vi "Hi-Tec_calibs.vi"(5 "Gas Line Name":string) -> (1 "Hi-Tec calib":T1={"Ref temp (deg C)"=0.0, "Ref Pres (mbars)"=0.0, "Density at calib conditions"=-0.0141, "Coefficients"=[]} {"Coefficients" format="%.2f"; "Density at calib conditions" format="%.4f"; "Ref Pres (mbars)" format="%.2f"; "Ref temp (deg C)" format="%.2f"}, 2 "Comments":string)   [LabVIEW 2015]
uses:
  Controls/Hi-Tec_calib.ctl
  Anemometry/Anemometry Sub Vis/Globals/Gas_management_global.vi
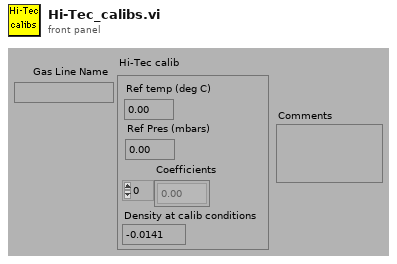
[diagram p1: front panel]
types:
  T1 = typedef "Hi-Tec_calib.ctl" = cluster{"Ref temp (deg C)":dbl, "Ref Pres (mbars)":dbl, "Density at calib conditions":dbl, "Coefficients":dbl[]}
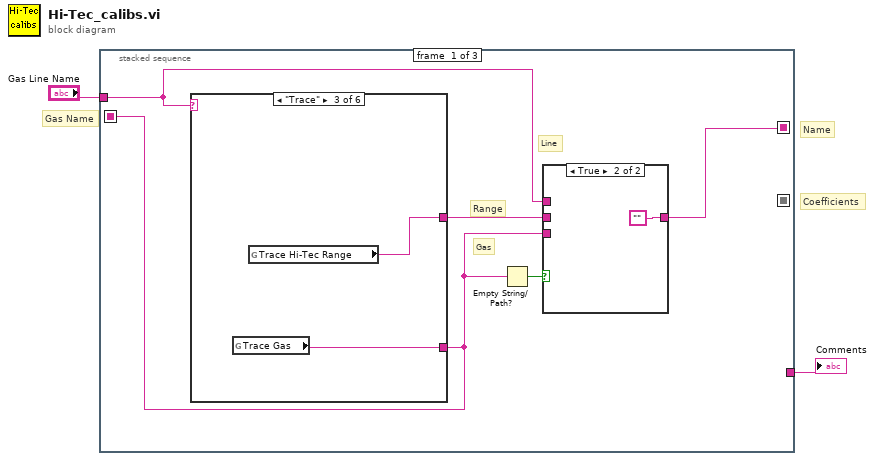
[diagram p0: block diagram]
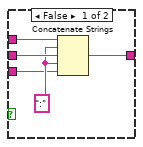
[diagram p2: hidden frame]
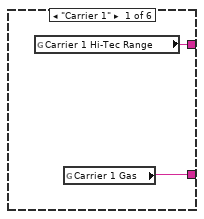
[diagram p3: hidden frame]
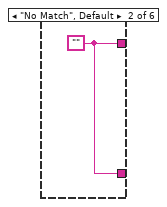
[diagram p4: hidden frame]
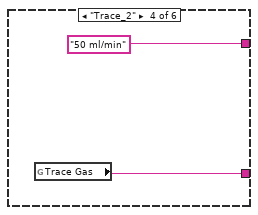
[diagram p5: hidden frame]
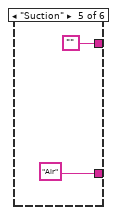
[diagram p6: hidden frame]
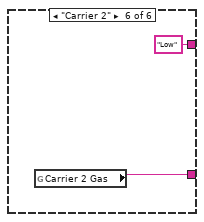
[diagram p7: hidden frame]
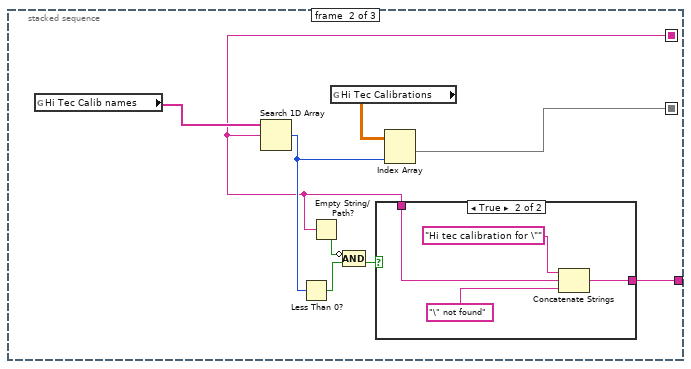
[diagram p8: hidden frame]
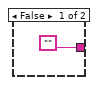
[diagram p9: hidden frame]
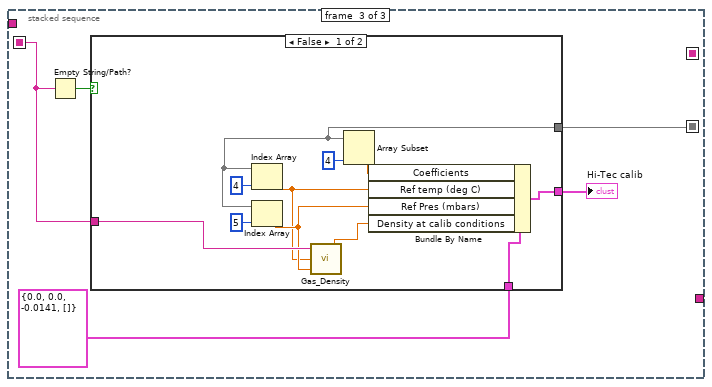
[diagram p10: hidden frame]
diagram:
  # "Name"
  # "Coefficients"
  # "Gas Name"
  n1 = stacked-sequence {
    seq-local: [w5 _ _] -> [_ _ w42]
    seq-local: [_ w31 _] -> [_ _ w39]
    seq-local: [w3 _ _] -> [_ w28 _]
    tunnel: "Gas Line Name" -> [w7 _ _]
    tunnel: [_ w29 _] -> w1
    frame #0 {
      # "Gas"
      # "Range"
      # "Line"
      n2 = case shown="\"Trace\"" w7 {
        tunnel: [w14 w16 w18 "50 ml/min" ("Trace Hi-Tec Range") "" "Low"] -> w6
        tunnel: [w15 w16 w17 w20 "Air" ("Carrier 2 Gas") w24] -> w5
        frame "Carrier 1" {
          n3 = global read "Gas_management_global.vi" "Carrier 1 Hi-Tec Range"() -> (w14:string)
          n4 = global read "Gas_management_global.vi" "Carrier 1 Gas"() -> (w15:string)
        }
        frame "No Match", Default {
          w16 = ""
        }
        frame "Trace" {
          n5 = global read "Gas_management_global.vi" "Trace Gas"() -> (w17:string)
          n6 = global read "Gas_management_global.vi" "Trace Hi-Tec Range"() -> (w18:string)
        }
        frame "Trace_2" {
          n7 = global read "Gas_management_global.vi" "Trace Gas"() -> (w20:string)
        }
        frame "Suction" {
        }
        frame "Carrier 2" {
          n8 = global read "Gas_management_global.vi" "Carrier 2 Gas"() -> (w24:string)
        }
      }
      n9 = Empty String/Path?(string/path=w5) -> (empty?=w4:bool)
      n10 = case shown="True" w4 {
        tunnel: w7 -> [w12 _]
        tunnel: w6 -> [w11 _]
        tunnel: w5 -> [w9 _]
        tunnel: [w8 ""] -> w3
        frame False {
          w10 = ":"
          n11 = Concatenate Strings(w12, w10, w11, w10, w9) -> (w8:string)
        }
        frame True {
        }
      }
    }
    frame #1 {
      n12 = global read "Gas_management_global.vi" "Hi Tec Calib names"() -> (w33:string[])
      n13 = Search 1D Array(1D array=w33, element=w28) -> (index of element=w30:i32)  [unwired: 1 out]
      n14 = Less Than 0?(x=w30) -> (x < 0?=w26:bool)
      n15 = Empty String/Path?(string/path=w28) -> (empty?=w27:bool)
      n16 = global read "Gas_management_global.vi" "Hi Tec Calibrations"() -> (w32:dbl[][])
      n17 = Compound Arithmetic op=AND(invert w27, w26) -> (w25:bool)
      n18 = case shown="True" w25 {
        tunnel: w28 -> [_ w37]
        tunnel: ["" w35] -> w29
        frame False {
        }
        frame True {
          n19 = Concatenate Strings("Hi tec calibration for \"", w37, "\" not found") -> (w35:string)
        }
      }
      n20 = Index Array(array=w32, index (col)=w30) -> (element=w31:dbl[])  [unwired: 1 in]
    }
    frame #2 {
      n21 = Empty String/Path?(string/path=w42) -> (empty?=w43:bool)
      n22 = case shown="False" w43 {
        tunnel: w42 -> [w53 _]
        tunnel: w39 -> [w46 _]
        tunnel: [w52 w55] -> w41
        tunnel: T1 {"Ref temp (deg C)"=0.0, "Ref Pres (mbars)"=0.0, "Density at calib conditions"=-0.0141, "Coefficients"=[]} ("Hi-Tec calib") -> [w51 w55]
        frame False {
          n23 = Index Array(array=w46, index=4) -> (element=w44:dbl)
          n24 = Index Array(array=w46, index=5) -> (element=w45:dbl)
          n25 = call "Gas_Density.vi"("Pressure (mbars)"=w45, "Temperature (deg C)"=w44, "Gas Name"=w53) -> ("Density Kg/m3"=w54:dbl)
          n26 = Array Subset(array=w46, length=4) -> (w49:dbl[])  [unwired: 1 in]
          n27 = Bundle By Name(cluster=w51, "Coefficients"=w49, "Ref temp (deg C)"=w44, "Ref Pres (mbars)"=w45, "Density at calib conditions"=w54) -> (w52:T1)
        }
        frame True {
        }
      }
      "Hi-Tec calib" <- w41
    }
  }
  "Comments" <- w1
